vi "Execute 7z bat.vi"(8 "error in (no error)":errorcluster, 11 "PostBuildSupport in":refnum<class "PostBuildSupport.lvclass">) -> (0 "error out":errorcluster, 3 "PostBuildSupport out":refnum<class "PostBuildSupport.lvclass">)   [LabVIEW 2016, in "PostBuildSupport.lvclass"]
uses:
  PostBuildSupport.lvclass
  PostBuildSupport.lvclass/PostBuildSupport.ctl
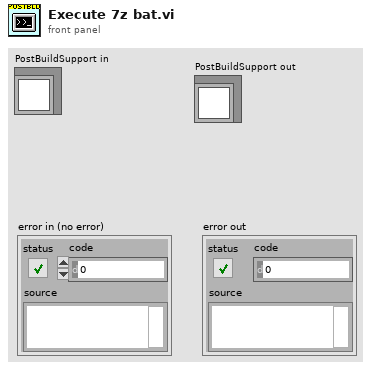
[diagram p1: front panel]
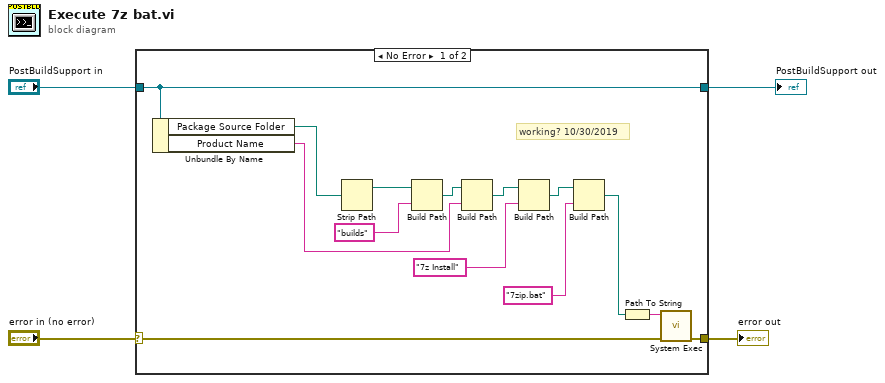
[diagram p0: block diagram]
diagram:
  n1 = case shown="No Error" "error in (no error)" {
    selector: "error in (no error)" -> [w12 w20]
    tunnel: [w18 w20] -> w1
    tunnel: "PostBuildSupport in" -> [w13 w19]
    tunnel: [w13 w19] -> w3
    frame No Error {
      # "working? 10/30/2019"
      n2 = Unbundle By Name(w13) -> ("Package Source Folder"=w17:path, "Product Name"=w14:string)
      n3 = Strip Path(path=w17) -> (stripped path=w8:path)  [unwired: 1 out]
      n4 = Build Path(base path=w8, name or relative path="builds") -> (appended path=w15:path)
      n5 = Build Path(base path=w15, name or relative path=w14) -> (appended path=w7:path)
      n6 = Build Path(base path=w7, name or relative path="7z Install") -> (appended path=w11:path)
      n7 = Build Path(base path=w11, name or relative path="7zip.bat") -> (appended path=w5:path)
      n8 = Path To String(path=w5) -> (string=w9:string)
      n9 = call <vilib>:"System Exec.vi"("error in (no error)"=w12, "command line"=w9) -> ("error out"=w18:errorcluster)  [unwired: 6 in, 3 out]
    }
    frame Error {
    }
  }
  "error out" <- w1
  "PostBuildSupport out" <- w3
